vi "remote co.vi"(1 "input":dbl) -> (0 "x*y":dbl)   [LabVIEW 2019]
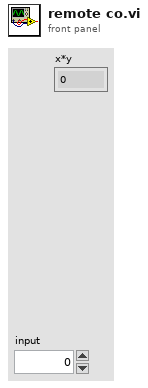
[diagram p1: front panel]
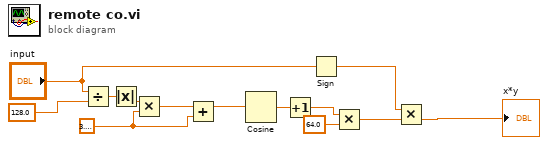
[diagram p0: block diagram]
diagram:
  w6 = 3.141592653589793
  n1 = Divide(x="input", y=128.0) -> (x/y=w13:dbl)
  n2 = Absolute Value(x=w13) -> (abs(x)=w8:dbl)
  n3 = Multiply(x=w8, y=w6) -> (x*y=w9:dbl)
  n4 = Add(x=w9, y=w6) -> (x+y=w7:dbl)
  n5 = Cosine(x=w7) -> (cos(x)=w12:dbl)
  n6 = Increment(x=w12) -> (x+1=w5:dbl)
  n7 = Sign(1:"input") -> (0:w1:dbl)
  n8 = Multiply(x=w5, y=64.0) -> (x*y=w10:dbl)
  n9 = Multiply(x=w1, y=w10) -> (x*y=→"x*y":dbl)
